vi "ship_battle_top.vi"() -> ()   [LabVIEW 2014]
panel:
  in  "Ring 6":u16(ring)=1
  in  "Ring 5":u16(ring)=2
  in  "Ring 4":u16(ring)=3
  out "Array 3":u16[][](array[ring])
  out "Array 2":u16[][](array[ring])
  in  "Array":u16[][](array[ring])=[[0, 0, 0, 0, 0, 0, 0, 0], [0, 0, 0, 0, 0, 0, 0, 0], [0, 0, 0, 0, 0, 0, 0, 0], [0, 0, 0, 0, 0, 0, 0, 0], [0, 0, 0, 0, 0, 0, 0, 0], [0, 0, 0, 0, 0, 0, 0, 0], [0, 0, 0, 0, 0, 0, 0, 0], [0, 0, 0, 0, 0, 0, 0, 0]]
  out "Miss":i32
  out "Hit":i32
  in  "Fire":bool
  in  "Fire Column":i32=2
  in  "Fire Raw":i32=1
  in  "Cluster":T1
  # "放置區"
  # "1             2              3             4              5              6             7              8"
  # "1"
  # "2"
  # "3"
  # "4"
  # "5"
  # "6"
  # "7"
  # "ship"
  # "Sea"
  # "hit"
  # "miss"
  # "8"
  # "遊玩區"
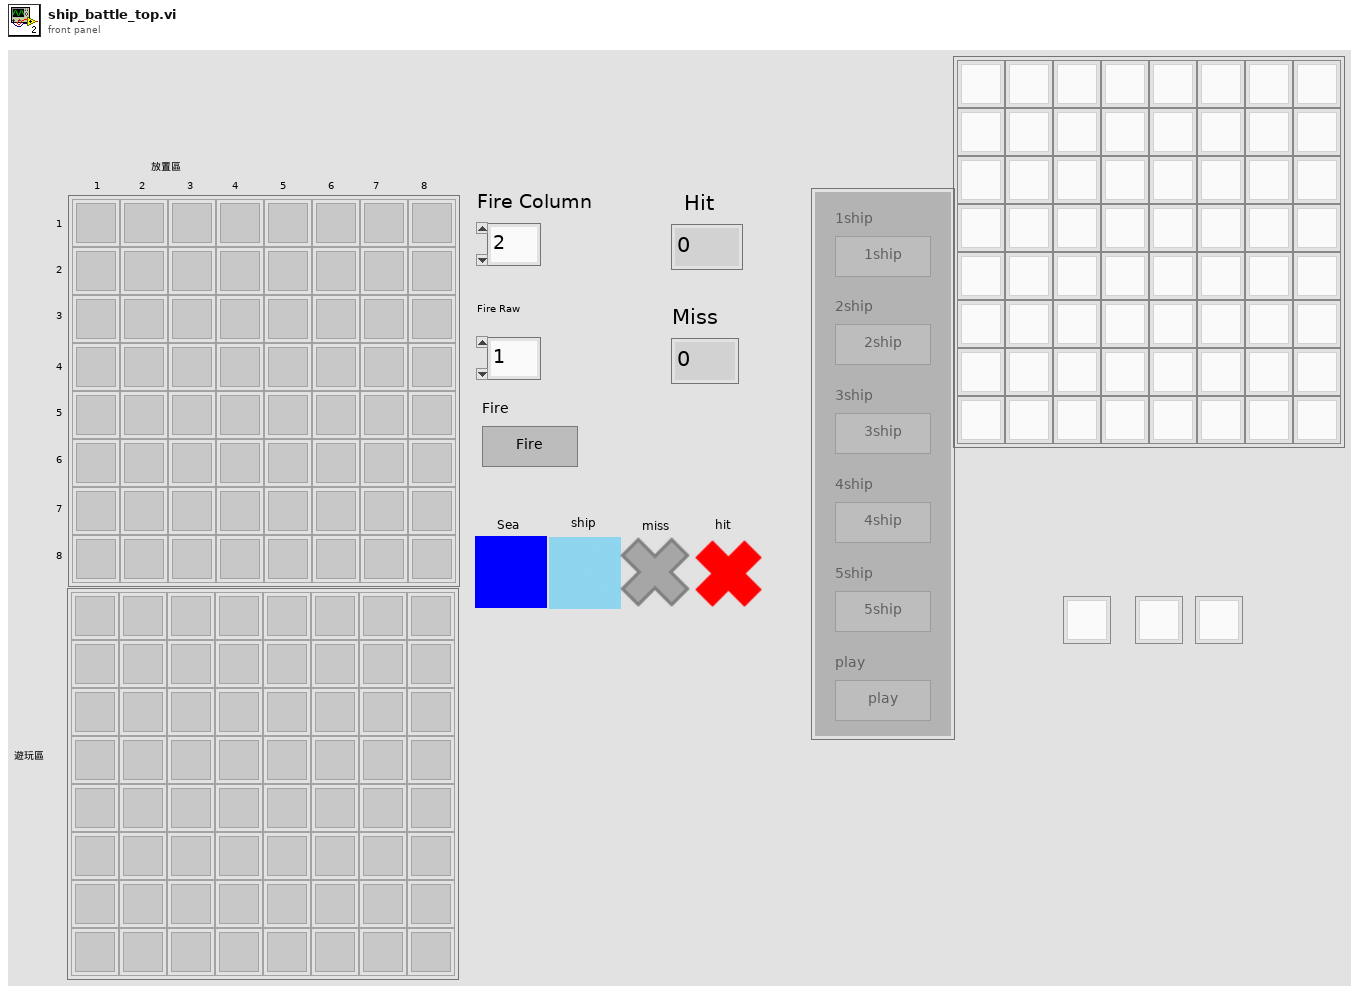
[diagram p1: front panel]
types:
  T1 = cluster{"1ship":bool, "2ship":bool, "3ship":bool, "4ship":bool, "5ship":bool, "play":bool}
  T2 = enum8{"Enabled", "Disabled", "Disabled and Grayed Out"}
  T3 = enum16{"wait", "1ship", "2ship", "3ship", "4ship", "5ship", "play"}
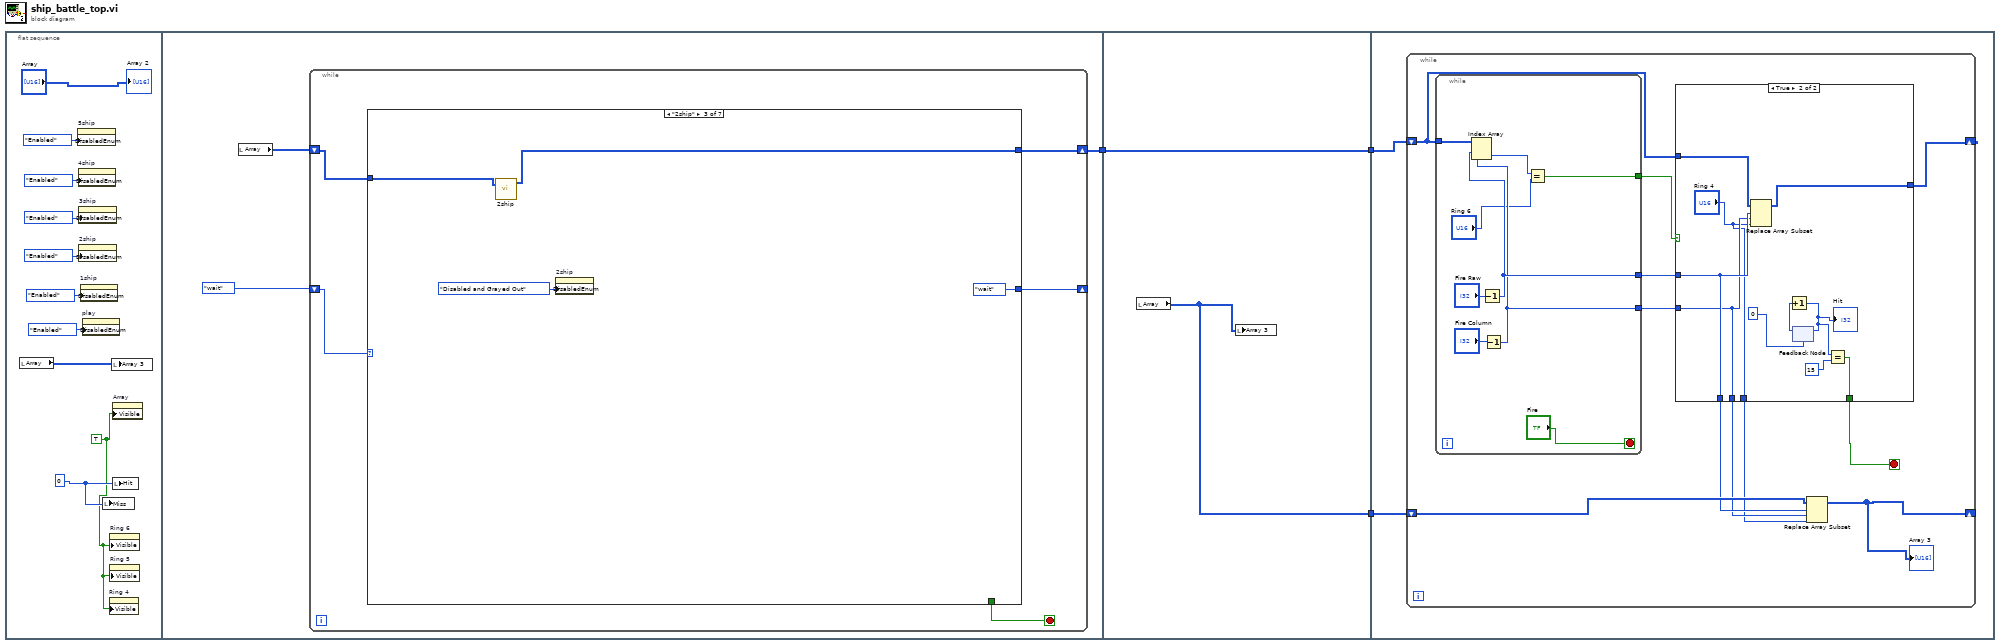
[diagram p0: block diagram]
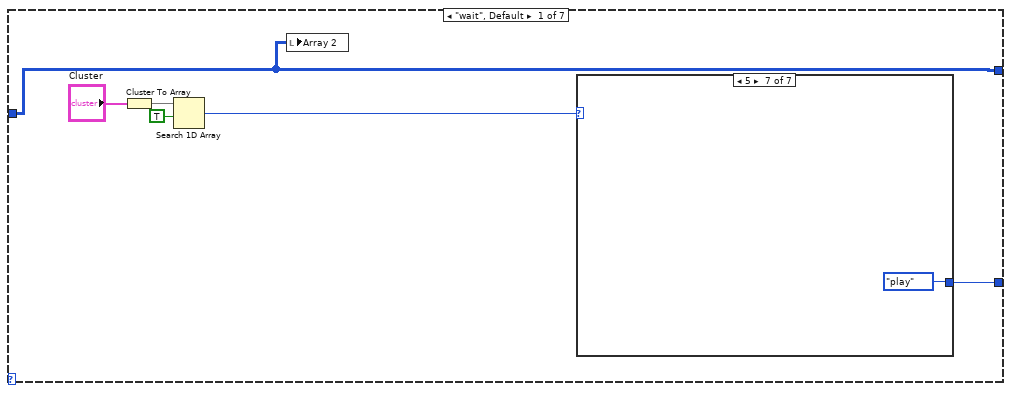
[diagram p2: hidden frame]
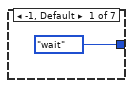
[diagram p3: hidden frame]
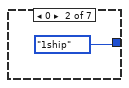
[diagram p4: hidden frame]
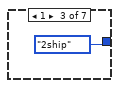
[diagram p5: hidden frame]
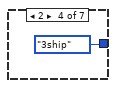
[diagram p6: hidden frame]
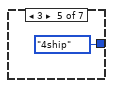
[diagram p7: hidden frame]
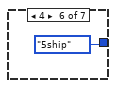
[diagram p8: hidden frame]
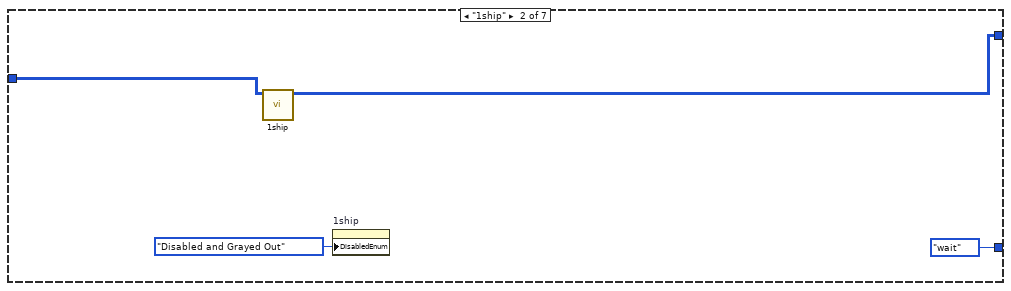
[diagram p9: hidden frame]
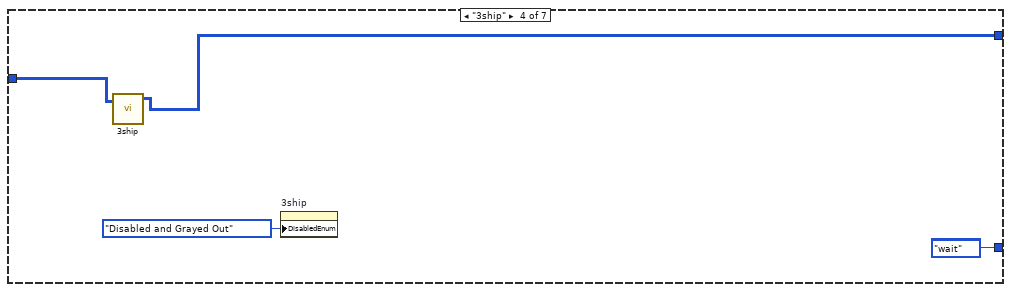
[diagram p10: hidden frame]
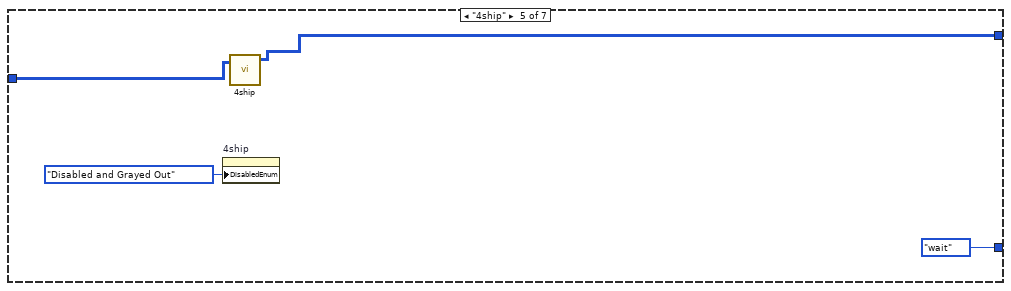
[diagram p11: hidden frame]
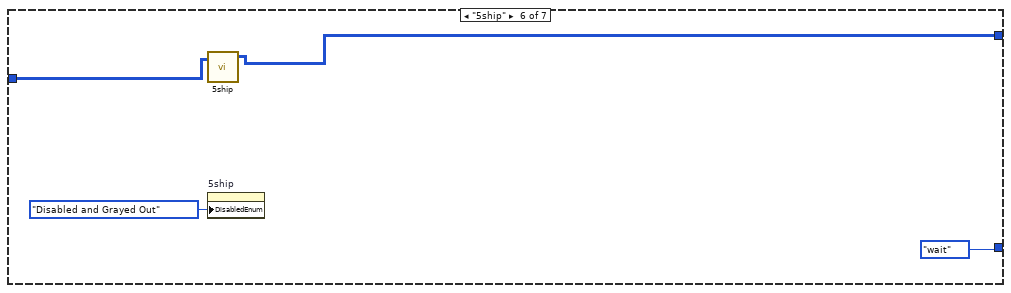
[diagram p12: hidden frame]
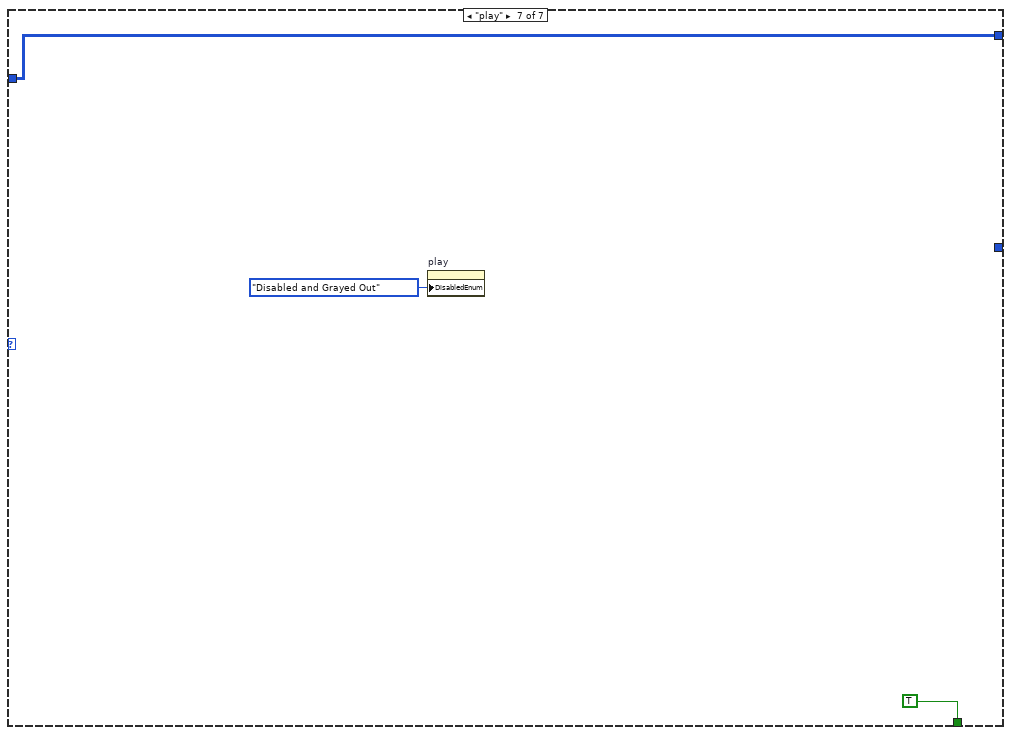
[diagram p13: hidden frame]
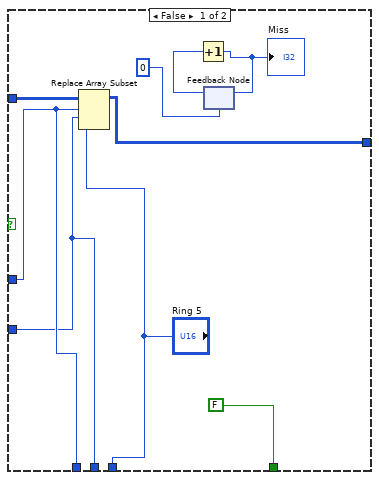
[diagram p14: hidden frame]
diagram:
  n1 = flat-sequence {
    tunnel: [w14] -> w3
    tunnel: w3 -> [w59]
    tunnel: [w59] -> w2
    tunnel: [w58] -> w1
    tunnel: w2 -> [w61]
    tunnel: w1 -> [w60]
    frame #0 {
      w6 = 0
      w4 = TRUE ("Visible")
      n2 = local read "Array"() -> (w7:u16[][])
      n3 = property on="5ship" class="Bool"("DisabledEnum"=T2."Enabled" ("Disabled")) -> ()  [unwired: 2 in, 2 out]
      n4 = property on="4ship" class="Bool"("DisabledEnum"=T2."Enabled" ("Disabled")) -> ()  [unwired: 2 in, 2 out]
      n5 = property on="3ship" class="Bool"("DisabledEnum"=T2."Enabled" ("Disabled")) -> ()  [unwired: 2 in, 2 out]
      n6 = property on="2ship" class="Bool"("DisabledEnum"=T2."Enabled" ("Disabled")) -> ()  [unwired: 2 in, 2 out]
      n7 = property on="1ship" class="Bool"("DisabledEnum"=T2."Enabled" ("Disabled")) -> ()  [unwired: 2 in, 2 out]
      n8 = property on="play" class="Bool"("DisabledEnum"=T2."Enabled" ("Disabled")) -> ()  [unwired: 2 in, 2 out]
      n9 = local write "Miss"(w6) -> ()
      n10 = property on="Ring 4" class="Ring (strict)"("Visible"=w4) -> ()  [unwired: 2 in, 2 out]
      n11 = property on="Ring 6" class="Ring (strict)"("Visible"=w4) -> ()  [unwired: 2 in, 2 out]
      n12 = property on="Ring 5" class="Ring (strict)"("Visible"=w4) -> ()  [unwired: 2 in, 2 out]
      n13 = local write "Array 3"(w7) -> ()
      n14 = property on="Array" class="Arr (strict)"("Visible"=w4) -> ()  [unwired: 2 in, 2 out]
      n15 = local write "Hit"(w6) -> ()
      "Array 2" <- "Array"
    }
    frame #1 {
      n16 = local read "Array"() -> (w15:u16[][])
      n17 = while {
        shift-right: [w20] -> _
        shift-left: T3."wait" -> [w21]
        shift-right: [w18] -> w14
        shift-left: w15 -> [w17]
        stop <- w19 stop-if-true
        n18 = case shown="\"2ship\"" w21 {
          tunnel: [w23 T3."wait" T3."wait" T3."wait" T3."wait" T3."wait" _] -> w20
          tunnel: [_ _ _ _ _ _ TRUE] -> w19
          tunnel: [w22 w37 w42 w44 w48 w52 w55] -> w18
          tunnel: w17 -> [w22 w38 w41 w43 w47 w51 w55]
          frame "wait", Default {
            n19 = Cluster To Array(cluster="Cluster") -> (array=w26:bool[])
            n20 = Search 1D Array(1D array=w26, element=TRUE) -> (index of element=w24:i32)  [unwired: 1 in]
            n21 = local write "Array 2"(w22) -> ()
            n22 = case shown="5" w24 {
              tunnel: [T3."wait" T3."1ship" T3."2ship" T3."3ship" T3."4ship" T3."5ship" T3."play"] -> w23
              frame -1, Default {
              }
              frame 0 {
              }
              frame 1 {
              }
              frame 2 {
              }
              frame 3 {
              }
              frame 4 {
              }
              frame 5 {
              }
            }
          }
          frame "1ship" {
            n23 = call "1ship.vi"("Array"=w38) -> ("Array 2"=w37:u16[][])  [unwired: 10 in]
            n24 = property on="1ship" class="Bool"("DisabledEnum"=T2."Disabled and Grayed Out" ("Disabled")) -> ()  [unwired: 2 in, 2 out]
          }
          frame "2ship" {
            n25 = call "2ship.vi"("Array"=w41) -> ("Array 2"=w42:u16[][])  [unwired: 3 in]
            n26 = property on="2ship" class="Bool"("DisabledEnum"=T2."Disabled and Grayed Out" ("Disabled")) -> ()  [unwired: 2 in, 2 out]
          }
          frame "3ship" {
            (unwired) T3."wait"
            n27 = call "3ship.vi"("Array"=w43) -> ("Array 2"=w44:u16[][])  [unwired: 3 in]
            n28 = property on="3ship" class="Bool"("DisabledEnum"=T2."Disabled and Grayed Out" ("Disabled")) -> ()  [unwired: 2 in, 2 out]
          }
          frame "4ship" {
            n29 = property on="4ship" class="Bool"("DisabledEnum"=T2."Disabled and Grayed Out" ("Disabled")) -> ()  [unwired: 2 in, 2 out]
            n30 = call "4ship.vi"("Array"=w47) -> ("Array 2"=w48:u16[][])  [unwired: 3 in]
          }
          frame "5ship" {
            n31 = call "5ship.vi"("Array"=w51) -> ("Array 2"=w52:u16[][])  [unwired: 3 in]
            n32 = property on="5ship" class="Bool"("DisabledEnum"=T2."Disabled and Grayed Out" ("Disabled")) -> ()  [unwired: 2 in, 2 out]
          }
          frame "play" {
            n33 = property on="play" class="Bool"("DisabledEnum"=T2."Disabled and Grayed Out" ("Disabled")) -> ()  [unwired: 2 in, 2 out]
          }
        }
      }
    }
    frame #2 {
      n34 = local read "Array"() -> (w58:u16[][])
      n35 = local write "Array 3"(w58) -> ()
    }
    frame #3 {
      n36 = while {
        shift-right: [w64] -> _
        shift-left: w61 -> [w71]
        shift-right: [w62] -> _
        shift-left: w60 -> [w68]
        stop <- w63 stop-if-true
        n37 = while {
          tunnel: w71 -> [w100]
          tunnel: [w96] -> w72
          tunnel: [w94] -> w70
          tunnel: [w93] -> w69
          stop <- "Fire" stop-if-true
          n38 = Decrement(x="Fire Raw") -> (x-1=w94:i32)
          n39 = Decrement(x="Fire Column") -> (x-1=w93:i32)
          n40 = Index Array(array=w100, index (row)=w94, index (col)=w93) -> (element=w97:u16)
          n41 = Equal?(x=w97, y="Ring 6") -> (x = y?=w96:bool)
        }
        n42 = case shown="True" w72 {
          tunnel: w71 -> [w81 w91]
          tunnel: w70 -> [w76 w85]
          tunnel: w69 -> [w75 w84]
          tunnel: [w77 w86] -> w64
          tunnel: [w76 w85] -> w67
          tunnel: [w75 w84] -> w66
          tunnel: ["Ring 5" "Ring 4"] -> w65
          tunnel: [FALSE ("stop") w83] -> w63
          frame False {
            n43 = Replace Array Subset(array=w81, new element="Ring 5", index (row)=w76, index (col)=w75) -> (w77:u16[][])
            n44 = feedback #1(0) -> (w79:i32)
            n45 = Increment(x=w79) -> (x+1=w80:i32)
            "Miss" <- w80
            n46 = feedback-in #1(w80) -> ()
          }
          frame True {
            n47 = Replace Array Subset(array=w91, new element="Ring 4", index (row)=w85, index (col)=w84) -> (w86:u16[][])
            n48 = feedback #2(0) -> (w88:i32)
            n49 = Increment(x=w88) -> (x+1=w87:i32)
            "Hit" <- w87
            n50 = feedback-in #2(w87) -> ()
            n51 = Equal?(x=w87, y=15) -> (x = y?=w83:bool)
          }
        }
        n52 = Replace Array Subset(array=w68, new element=w65, index (row)=w67, index (col)=w66) -> (w62:u16[][])
        "Array 3" <- w62
      }
    }
  }
